vi "6602_Trigger_Dev3.vi"(10 "Experiment State":T1={"Send Trigger 3"=FALSE, "error"={"status"=FALSE, "code"=0, "source"=""}, "Digitizer DAQmx Tasks"={"TaskArray"=[]}, "Digitizer Settings"={"6133 Digitizer Channels"=[], "Global Edge Type"=10280, "Total Samples"=[], "Pre-Trigger Samples"=[], "Sample Rate"=[], "Trigger Sources"=[], "Voltage Ranges"=[], "Channel Names"=[], "Active"=[], "Samples to remove"=[], "Start Time"=[], "End Time"=[]}, "Synchronization Settings"={"Position"="PXI1Slot2", "source terminal"="GlobalSoftwareTrigger"}, "Digitizer Data"=[], "Next Shot#"="0", "System Message"="", "User Shot Notes"="", "Timing Settings"={"Timing Card Settings"=[], "Timing Channel Settings"=[[{"Delay (s)"=2.559999942779541, "Pulse width (s)"=0.009999999776482582, "Active"=TRUE, "Channel Name"="Fiber 8", "counter"="PXI1Slot8/ctr7"}]]}} {"Timing Settings"."Timing Channel Settings"."Pulse width (s)" format="%.3p"; "Timing Settings"."Timing Channel Settings"."Delay (s)" format="%.3p"; "Digitizer Settings"."Sample Rate" format="%#_3p"; "Digitizer Settings"."Global Edge Type" items=["Rising"=10280, "Falling"=10171]}, 11 "Dev Select":enum16{"Dev 8", "Dev 9"}(ring)) -> (2 "Experiment State":T1={"Send Trigger 3"=FALSE, "error"={"status"=FALSE, "code"=0, "source"=""}, "Digitizer DAQmx Tasks"={"TaskArray"=[]}, "Digitizer Settings"={"6133 Digitizer Channels"=[], "Global Edge Type"=10280, "Total Samples"=[], "Pre-Trigger Samples"=[], "Sample Rate"=[], "Trigger Sources"=[], "Voltage Ranges"=[], "Channel Names"=[], "Active"=[], "Samples to remove"=[], "Start Time"=[], "End Time"=[]}, "Synchronization Settings"={"Position"="PXI1Slot2", "source terminal"="GlobalSoftwareTrigger"}, "Digitizer Data"=[], "Next Shot#"="0", "System Message"="", "User Shot Notes"="", "Timing Settings"={"Timing Card Settings"=[], "Timing Channel Settings"=[[{"Delay (s)"=2.559999942779541, "Pulse width (s)"=0.009999999776482582, "Active"=TRUE, "Channel Name"="Fiber 8", "counter"="PXI1Slot8/ctr7"}]]}} {"Timing Settings"."Timing Channel Settings"."Pulse width (s)" format="%.3p"; "Timing Settings"."Timing Channel Settings"."Delay (s)" format="%.3p"; "Digitizer Settings"."Sample Rate" format="%#_3p"; "Digitizer Settings"."Global Edge Type" items=["Rising"=10280, "Falling"=10171]})   [LabVIEW 2013]
uses:
  <vilib>/DAQmx/create/channels.llb/DAQmx Create Channel (CO-Pulse Generation-Time).vi
  <vilib>/DAQmx/configure/timing.llb/DAQmx Timing (Implicit).vi
  <vilib>/DAQmx/configure/trigger.llb/DAQmx Start Trigger (Digital Edge).vi
  Controls/ExperimentStateCluster.ctl
panel:
  # "Channel Settings"
  # "Card Wide Settings"
  # "Channel Settings"
  # "Card Wide Settings"
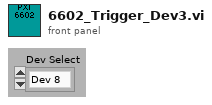
[diagram p1: front panel]
types:
  T1 = typedef "ExperimentStateCluster.ctl" = cluster{"Send Trigger 3":bool, "error":errorcluster, "Digitizer DAQmx Tasks":cluster{"TaskArray":refnum<k21>[]}, "Digitizer Settings":cluster{"6133 Digitizer Channels":tag[][], "Global Edge Type":i32, "Total Samples":i32[], "Pre-Trigger Samples":u32[], "Sample Rate":dbl[], "Trigger Sources":tag[], "Voltage Ranges":dbl[][], "Channel Names":string[][], "Active":bool[][], "Samples to remove":u32[], "Start Time":dbl[], "End Time":dbl[]}, "Synchronization Settings":cluster{"Position":refnum<k15>, "source terminal":string}, "Digitizer Data":waveform(dbl)[][], "Next Shot#":string, "System Message":string, "User Shot Notes":string, "Timing Settings":cluster{"Timing Card Settings":cluster{"Slot 8 Trigger Source":tag, "Clock Source":tag, "Trigger Channel Tasks":refnum<k21>[]}[], "Timing Channel Settings":cluster{"Delay (s)":dbl, "Pulse width (s)":dbl, "Active":bool, "Channel Name":string, "counter":tag}[][]}}
  T2 = cluster{"Delay (s)":dbl, "Pulse width (s)":dbl, "Active":bool, "Channel Name":string, "counter":tag}[]
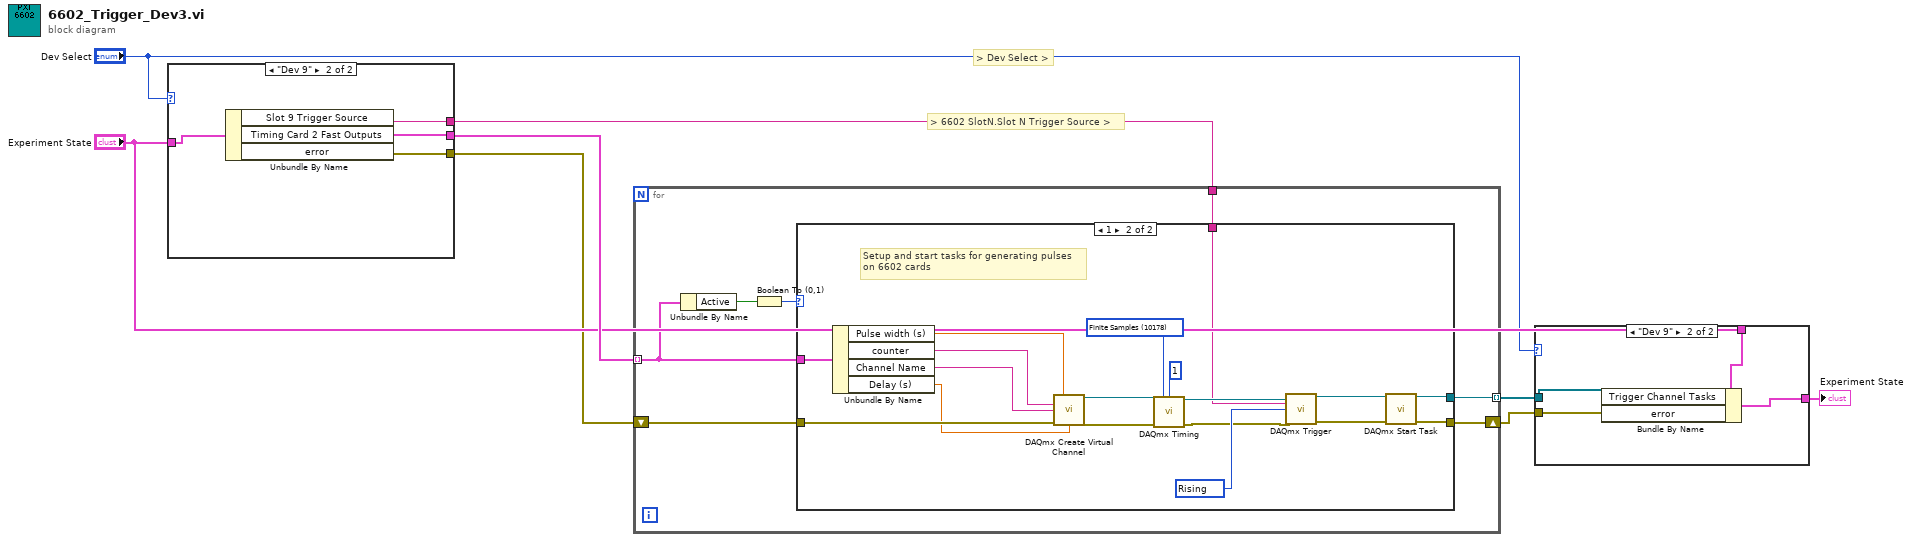
[diagram p0: block diagram]
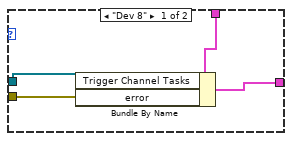
[diagram p2: hidden frame]
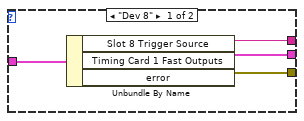
[diagram p3: hidden frame]
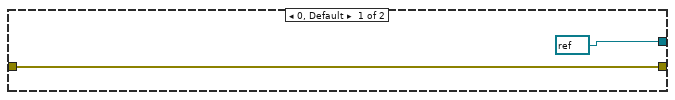
[diagram p4: hidden frame]
diagram:
  # "> Dev Select >"
  # "> 6602 SlotN.Slot N Trigger Source >"
  n1 = case shown="\"Dev 9\"" "Dev Select" {
    tunnel: "Experiment State" -> [w12 w16]
    tunnel: [w11 w15] -> w3
    tunnel: [w10 w14] -> w8
    tunnel: [w9 w13] -> w7
    frame "Dev 8" {
      n2 = Unbundle By Name(w12) -> ("Slot 8 Trigger Source"=w10:tag, "Timing Card 1 Fast Outputs"=w9:T2, "error"=w11:errorcluster)
    }
    frame "Dev 9" {
      n3 = Unbundle By Name(w16) -> ("Slot 9 Trigger Source"=w14:tag, "Timing Card 2 Fast Outputs"=w13:T2, "error"=w15:errorcluster)
    }
  }
  n4 = for {
    tunnel: w7 -> [w19] mode=indexing
    tunnel: w8 -> [w21]
    shift-right: [w18] -> w1
    shift-left: w3 -> [w17]
    tunnel: [w23] -> w2 mode=indexing
    n5 = Unbundle By Name(w19) -> ("Active"=w20:bool)
    n6 = Boolean To (0,1)(Boolean=w20) -> (0, 1=w22:i16)
    n7 = case shown="1" w22 {
      tunnel: [refnum<k21> refnum ("task out") w33] -> w23
      tunnel: [w25 w32] -> w18
      tunnel: w21 -> [_ w26]
      tunnel: w19 -> [_ w43]
      tunnel: w17 -> [w25 w40]
      frame 0, Default {
      }
      frame 1 {
        w29 = 10280 items=["Rising"=10280, "Falling"=10171] ("Start.DigEdge.Edge")
        w34 = 10178 items=["Finite Samples"=10178, "Continuous Samples"=10123, "Hardware Timed Single Point"=12522] ("sample mode")
        # "Setup and start tasks for generating pulses\non 6602 cards"
        n8 = Unbundle By Name(w43) -> ("Pulse width (s)"=w39:dbl, "counter"=w42:tag, "Channel Name"=w41:string, "Delay (s)"=w38:dbl)
        n9 = call-poly <vilib>:"DAQmx Create Virtual Channel.vi"("high time"=w39, "counter"=w42, "name to assign"=w41, "error in"=w40, "initial delay"=w38) -> ("task out"=w37:refnum<k21>, "error out"=w36:errorcluster)  [unwired: 4 in, 5 out]
        n10 = call-poly <vilib>:"DAQmx Timing.vi"("task/channels in"=w37, "sample mode"=w34, "samples per channel"=1, "error in"=w36) -> ("task out"=w27:refnum<k21>, "error out"=w28:errorcluster)  [unwired: 10 in]
        n11 = call-poly <vilib>:"DAQmx Trigger.vi"("task/channels in"=w27, "source"=w26, "edge"=w29, "error in"=w28) -> ("task out"=w31:refnum<k21>, "error out"=w30:errorcluster)  [unwired: 10 in]
        n12 = call <vilib>:"DAQmx Start Task.vi"("task/channels in"=w31, "error in"=w30) -> ("task out"=w33:refnum<k21>, "error out"=w32:errorcluster)  [unwired: 12 in]
      }
    }
  }
  n13 = case shown="\"Dev 9\"" "Dev Select" {
    tunnel: w2 -> [w44 w48]
    tunnel: [w47 w51] -> w6
    tunnel: "Experiment State" -> [w46 w50]
    tunnel: w1 -> [w45 w49]
    frame "Dev 8" {
      n14 = Bundle By Name(cluster=w46, "Trigger Channel Tasks"=w44, "error"=w45) -> (w47:T1)
    }
    frame "Dev 9" {
      n15 = Bundle By Name(cluster=w50, "Trigger Channel Tasks"=w48, "error"=w49) -> (w51:T1)
    }
  }
  "Experiment State" <- w6
